vi "Configure Auto Polarity Control.vi"(8 "error in (no error)":errorcluster, 10 "Auto Polarity Control (F:Disable)":bool, 11 "VISA resource name":refnum<visa-resource-name>) -> (0 "error out":errorcluster, 3 "VISA resource name out":refnum<visa-resource-name>)   [LabVIEW 2017, in "Agilent E4980.lvlib"]
doc: "The automatic bias polarity control function is useful when testing a varactor diode. The instrument identifies the connection state of the diode using an internal bias (approx. 1 V), then the instrument internally controls the DC bias polarity so that a reverse bias is applied to the diode.\n\n<B>Notes:</B>\n(1) This is valid only when your instrument installs <B>Option 001</B> (Power and DC Bias enhancement)."
uses:
  Agilent E4980.lvlib
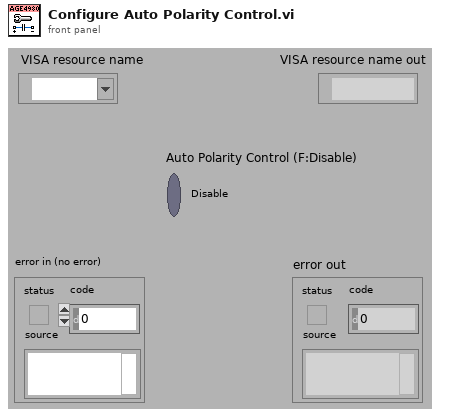
[diagram p1: front panel]
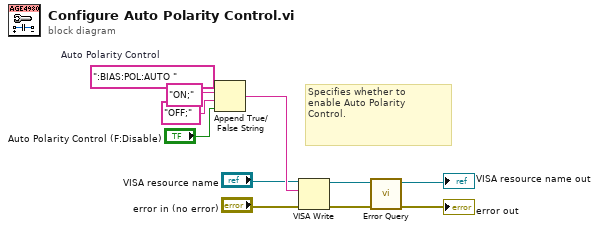
[diagram p0: block diagram]
diagram:
  w11 = ":BIAS:POL:AUTO "  # Auto Polarity Control
  # "Specifies whether to\nenable Auto Polarity\nControl."
  n1 = Append True/False String(1:"Auto Polarity Control (F:Disable)", 2:"OFF;" ("false string"), 3:"ON;" ("true string"), 4:w11) -> (0:w9:string)
  n2 = VISA Write(VISA resource name="VISA resource name", write buffer=w9, error in (no error)="error in (no error)") -> (VISA resource name out=w8:refnum<visa-resource-name>, error out=w7:errorcluster)  [unwired: 1 out]
  n3 = call "Error Query.vi"("error in (no error)"=w7, "VISA resource name"=w8) -> ("error out"=→"error out":errorcluster, "VISA resource name out"=→"VISA resource name out":refnum<visa-resource-name>)  [unwired: 6 in, 2 out]
